vi "aft_xmpl_Compute Speed from Tach Signal.vi"(9 "Threshold":dbl=2.0, 10 "pulse/cycle":i32=2, 11 "Tach":dbl) -> (2 "Speed Available?":bool, 3 "speed":dbl)   [LabVIEW 2019]
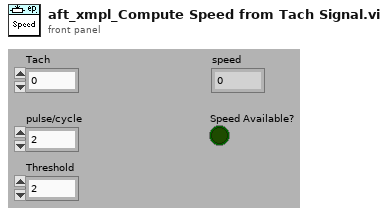
[diagram p1: front panel]
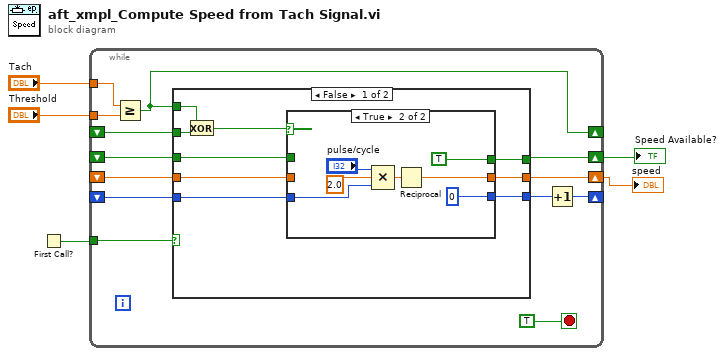
[diagram p0: block diagram]
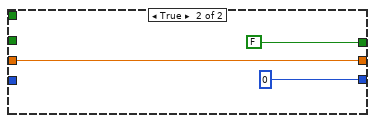
[diagram p3: hidden frame]
diagram:
  n1 = First Call?() -> (First Call?: T/F=w4:bool)
  n2 = while {
    tunnel: "Tach" -> [w10]
    shift-right: [w9] -> _
    shift-left: _ -> [w8]
    shift-right: [w17] -> _
    shift-left: _ -> [w16]
    tunnel: w4 -> [w7]
    shift-right: [w14] -> w3
    shift-left: _ -> [w13]
    shift-right: [w12] -> w2
    shift-left: _ -> [w11]
    tunnel: "Threshold" -> [w6]
    stop <- TRUE stop-if-true
    n3 = Greater Or Equal?(x=w10, y=w6) -> (x >= y?=w9:bool)
    n4 = case shown="False" w7 {
      tunnel: w9 -> [w27 _]
      tunnel: w16 -> [w26 _]
      tunnel: [w25 0] -> w15
      tunnel: [w24 FALSE] -> w12
      tunnel: [w23 w38] -> w14
      tunnel: w13 -> [w22 w38]
      tunnel: w11 -> [w21 _]
      tunnel: w8 -> [w20 _]
      frame False {
        n5 = Exclusive Or(1:w20, 2:w27) -> (0:w19:bool)
        n6 = case shown="True" w19 {
          tunnel: w26 -> [w30 w33]
          tunnel: [w30 0] -> w25
          tunnel: [w28 TRUE] -> w24
          tunnel: [w29 w31] -> w23
          tunnel: w22 -> [w29 _]
          tunnel: w21 -> [w28 _]
          frame False {
          }
          frame True {
            n7 = Compound Arithmetic op=MULTIPLY("pulse/cycle", 2.0 ("y"), w33) -> (w32:dbl)
            n8 = Reciprocal(x=w32) -> (1/x=w31:dbl)
          }
        }
      }
      frame True {
      }
    }
    n9 = Increment(x=w15) -> (x+1=w17:i32)
  }
  "speed" <- w3
  "Speed Available?" <- w2
